vi "PDE Rendering.vi"   [LabVIEW 2020, in "NI_PDE.lvlib"]
doc: "Renders the solution of the partial differential equation. You must manually select the polymorphic instance to use."
uses:
  <vilib>/gmath/NI_PDE.lvlib
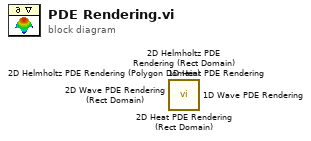
[diagram p0: block diagram]
diagram:
  n1 = call <vilib>:"2D Heat PDE Rendering (Rect Domain).vi"() -> ()  [unwired: 11 in, 5 out]
  n2 = call <vilib>:"1D Heat PDE Rendering.vi"() -> ()  [unwired: 11 in, 5 out]
  n3 = call <vilib>:"2D Wave PDE Rendering (Rect Domain).vi"() -> ()  [unwired: 11 in, 5 out]
  n4 = call <vilib>:"1D Wave PDE Rendering.vi"() -> ()  [unwired: 11 in, 5 out]
  n5 = call <vilib>:"2D Helmholtz PDE Rendering (Rect Domain).vi"() -> ()  [unwired: 11 in, 5 out]
  n6 = call <vilib>:"2D Helmholtz PDE Rendering (Polygon Domain).vi"() -> ()  [unwired: 12 in, 4 out]
